vi "ble_parse_scan_response.vi"(11 "Scan Response Data":u8[](array[numeric]) format="%02x") -> (3 "Array Scan Response":string[](array[string]))   [LabVIEW 2015]
uses:
  type_def/advertising_package_type.ctl
  type_def/address_type.ctl
panel:
  out "Friendly Name":string
  out "RSSI string":string
  out "Addvertiser Address Type":string
  in  "Address Type":T1 items=["Public", "Random"]
  out "MAC string OUT colon":string
  out "Advertising Package Type String":string
  in  "Advertising Package Type":T2 items=["Connectable Advertisement packet"=0, "Non Connectable Advertisement packet"=2, "Scan response packet"=4, "Discoverable advertisement packet"=6]
  out "RSSI (dBm)":i8
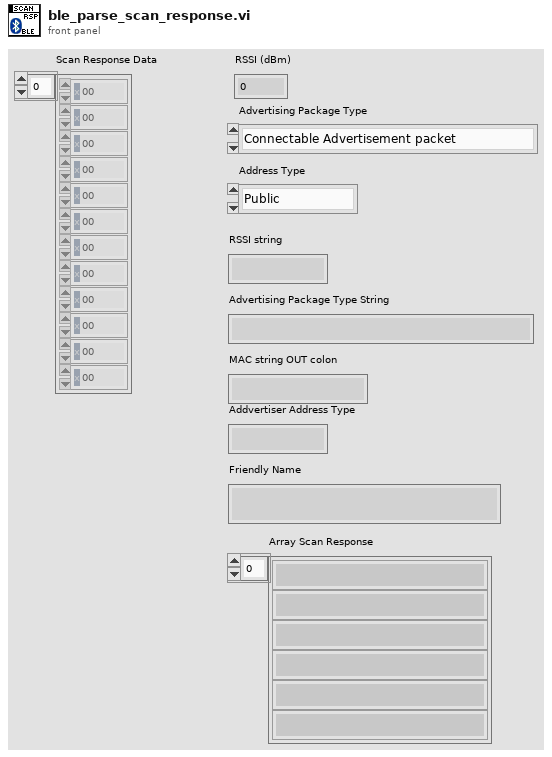
[diagram p1: front panel]
types:
  T1 = typedef "address_type.ctl" = u8
  T2 = typedef "advertising_package_type.ctl" = u8
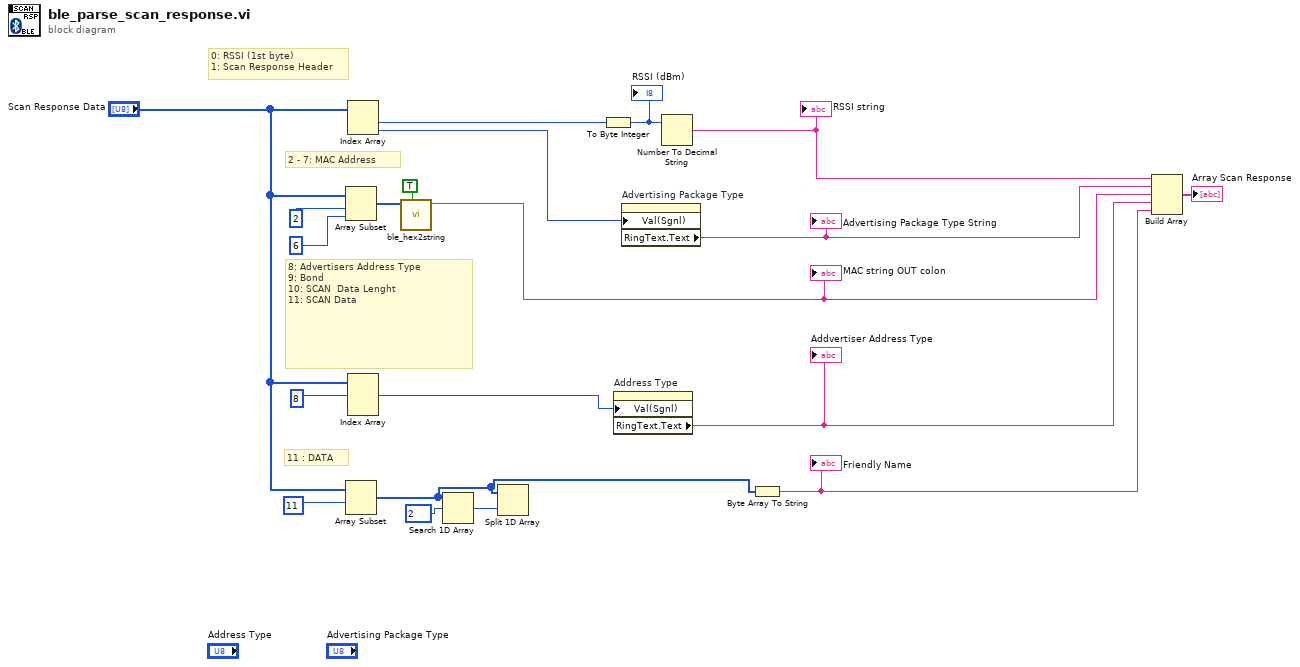
[diagram p0: block diagram]
diagram:
  # "11 : DATA"
  # "8: Advertisers Address Type\n9: Bond\n10: SCAN  Data Lenght\n11: SCAN Data"
  # "2 - 7: MAC Address"
  # "0: RSSI (1st byte)\n1: Scan Response Header"
  n1 = Array Subset(array="Scan Response Data", index=2, length=6) -> (w5:u8[])
  n2 = Array Subset(array="Scan Response Data", index=11 ("length")) -> (w1:u8[])  [unwired: 1 in]
  n3 = Index Array(array="Scan Response Data") -> (element #1=w20:u8, element #2=w14:u8)  [unwired: 2 in]
  n4 = Index Array(array="Scan Response Data", index #1=8 ("length")) -> (element #1=w13:u8)  [unwired: 2 in, 2 out]
  n5 = call "ble_hex2string.vi"("colon?(false)"=TRUE, "Byte Array IN (index0 LS byte)"=w5) -> ("HEX string OUT"=w4:string)  [unwired: 9 in]
  "MAC string OUT colon" <- w4
  n6 = Search 1D Array(1D array=w1, element=u8 2) -> (index of element=w8:i32)  [unwired: 1 in]
  n7 = Split 1D Array(array=w1, index=w8) -> ()  [unwired: 2 out]
  n8 = To Byte Integer(number=w20) -> (8bit integer=w17:i8)
  "RSSI (dBm)" <- w17
  n9 = property on="Address Type" class="Ring (엄격한)"("Val(Sgnl)"=w13) -> ("RingText.Text"=w10:string)  [unwired: 2 in, 2 out]
  "Addvertiser Address Type" <- w10
  n10 = property on="Advertising Package Type" class="Ring (엄격한)"("Val(Sgnl)"=w14) -> ("RingText.Text"=w11:string)  [unwired: 2 in, 2 out]
  "Advertising Package Type String" <- w11
  n11 = Number To Decimal String(number=w17) -> (decimal integer string=w12:string)  [unwired: 1 in]
  "RSSI string" <- w12
  n12 = Byte Array To String(unsigned byte array=w1) -> (string=w7:string)
  "Friendly Name" <- w7
  n13 = Build Array(w12, w11, w4, w10, w7) -> (→"Array Scan Response":string[])
